vi "driveShifterStateMachine.vi"(11 "Drive Shift State":T1=enum."High") -> ()   [LabVIEW 2018]
uses:
  driveShiftEnum.ctl
  <vilib>/Rock Robotics/WPI/Solenoid/WPI_SolenoidValue.ctl
  <vilib>/Rock Robotics/WPI/Solenoid/WPI_SolenoidSetEnum.vi
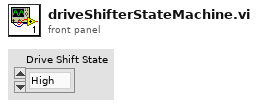
[diagram p1: front panel]
types:
  T1 = typedef "driveShiftEnum.ctl" = enum16{"Low", "High"}
  T2 = typedef "WPI_SolenoidValue.ctl" = enum16{"Off", "On", "Forward", "Reverse"}
  T3 = typedef "WPI_SolenoidDevRef.ctl" = cluster{"DevStatus":errorcluster, "Pneumatics Control Module":u8, "Forward Solenoid Channel":T4, "Reverse Solenoid Channel":T4}
  T4 = typedef "WPI_SolenoidChannel.ctl" = enum8{"Solenoid 0", "Solenoid 1", "Solenoid 2", "Solenoid 3", "Solenoid 4", "Solenoid 5", "Solenoid 6", "Solenoid 7", "Invalid"}
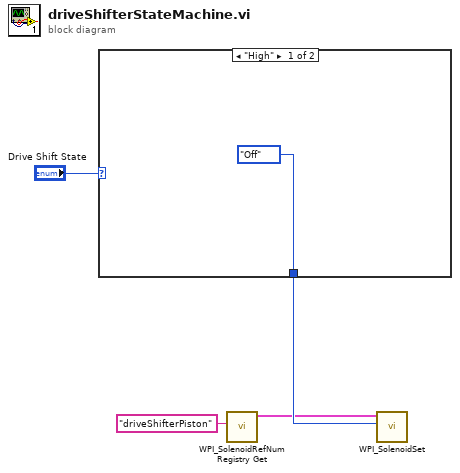
[diagram p0: block diagram]
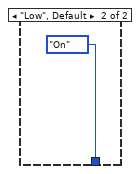
[diagram p2: hidden frame]
diagram:
  n1 = case shown="\"High\"" "Drive Shift State" {
    tunnel: [WPI_SolenoidValue."Off" ("Value") WPI_SolenoidValue."On" ("Value")] -> w3
    frame "High" {
    }
    frame "Low", Default {
    }
  }
  n2 = call <vilib>:"WPI_SolenoidRefNum Registry Get.vi"("refnum name"="driveShifterPiston") -> ("SolenoidDevRef"=w2:T3)  [unwired: 9 in, 1 out]
  n3 = call-poly <vilib>:"WPI_SolenoidSet.vi"("Value"=w3, "SolenoidDevRef"=w2) -> ()  [unwired: 8 in, 2 out]
